vi "Initialize Save Images VI.vi"(8 "error in (no error)":errorcluster, 11 "Channel in":refnum<class "Channel.lvclass">) -> (0 "error out":errorcluster, 3 "Channel out":refnum<class "Channel.lvclass">)   [LabVIEW 2018, in "Channel.lvclass"]
doc: "Run the VI responsible for saving the images"
uses:
  Channel.lvclass
  Channel.lvclass/Channel.ctl
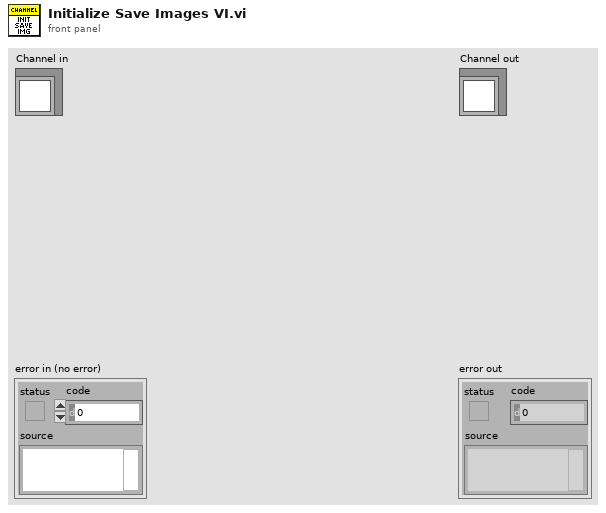
[diagram p1: front panel]
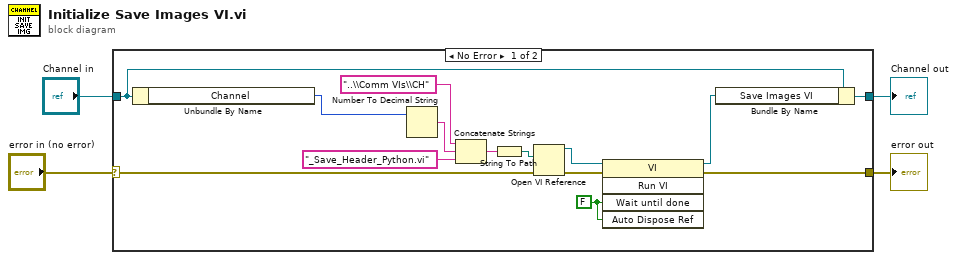
[diagram p0: block diagram]
diagram:
  n1 = case shown="No Error" "error in (no error)" {
    selector: "error in (no error)" -> [w9 w20]
    tunnel: [w14 w20] -> w3
    tunnel: [w6 w19] -> w1
    tunnel: "Channel in" -> [w7 w19]
    frame No Error {
      w17 = FALSE ("Wait Until Done")
      n2 = Unbundle By Name(w7) -> ("Channel"=w8:u8)
      n3 = Number To Decimal String(number=w8) -> (decimal integer string=w15:string)  [unwired: 1 in]
      n4 = Concatenate Strings("..\\Comm VIs\\CH" ("name or relative path"), w15, "_Save_Header_Python.vi" ("name or relative path")) -> (w11:string)
      n5 = String To Path(string=w11) -> (path=w12:path)
      n6 = Open VI Reference(vi path=w12, error in (no error)=w9) -> (vi reference=w18:refnum<vi>, error out=w10:errorcluster)  [unwired: 4 in]
      n7 = invoke class="VI" method="Run VI"(reference=w18, error in=w10, "Wait until done"=w17, "Auto Dispose Ref"=w17) -> (reference out=w5:refnum<vi>, error out=w14:errorcluster)  [unwired: 1 in, 3 out]
      n8 = Bundle By Name(cluster=w7, "Save Images VI"=w5) -> (w6:refnum<class "Channel.lvclass">)
    }
    frame Error {
    }
  }
  "error out" <- w3
  "Channel out" <- w1
